vi "crop_test.vi"() -> ()   [LabVIEW 2017]
uses:
  Vision.lvlib
panel:
  in  "bottom":i32=40
  in  "top":i32=20
  in  "right":i32=40
  in  "left":i32=20
  in  "File Path":path=path "C:/Users/Caleb/Desktop/obama.jpg"
  out "error out":errorcluster
  out "Image":T1(plugin-control)
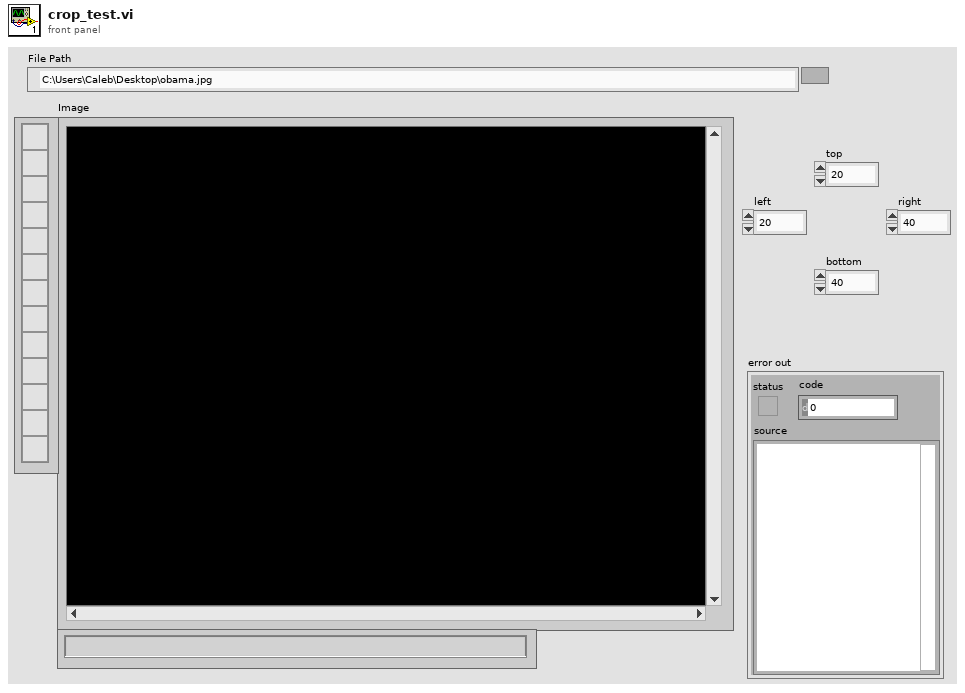
[diagram p1: front panel]
types:
  T1 = typedef "IMAQ Image.ctl" = refnum<image>
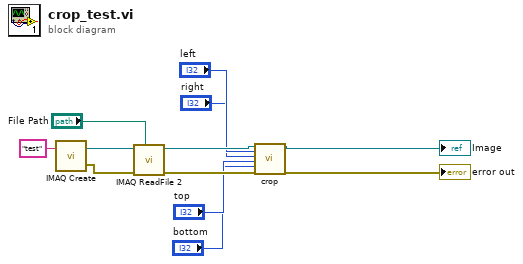
[diagram p0: block diagram]
diagram:
  n1 = call "IMAQ Create"("Image Name"="test") -> ("New Image"=w12:T1, "error out"=w10:errorcluster)  [unwired: 4 in]
  n2 = call "IMAQ ReadFile 2"("File Path"="File Path", "error in (no error)"=w10, "Image"=w12) -> ("error out"=w7:errorcluster, "Image Out"=w8:T1)  [unwired: 4 in, 3 out]
  n3 = call "crop.vi"("Image in"=w8, "left"="left", "right"="right", "top"="top", "bottom"="bottom", "error in (no error)"=w7) -> ("Image out"=→"Image":T1, "error out"=→"error out":errorcluster)  [unwired: 12 in]
